vi "RNG WriteState.vi"(8 "error in (no error)":errorcluster, 10 "State":u64, 11 "RNG in":refnum<class "RNG.lvclass">) -> (0 "error out":errorcluster, 3 "RNG out":refnum<class "RNG.lvclass">)   [LabVIEW 2020, in "OpenLvVision_OpenCv.lvlib" / "RNG.lvclass"]
doc: "Write the state to the rng object."
uses:
  RNG.lvclass
  _LvHelpers/EdvrObject/EdvrObject.lvclass
  Dlls/OlvOpenCvWrapper.dll
  C:/Users/lukas/Downloads/OpenLvVision_OpenCv/SourceCode/LabView/OpenLvVision_OpenCv/_LvHelpers/EdvrObject/EdvrObject.lvclass
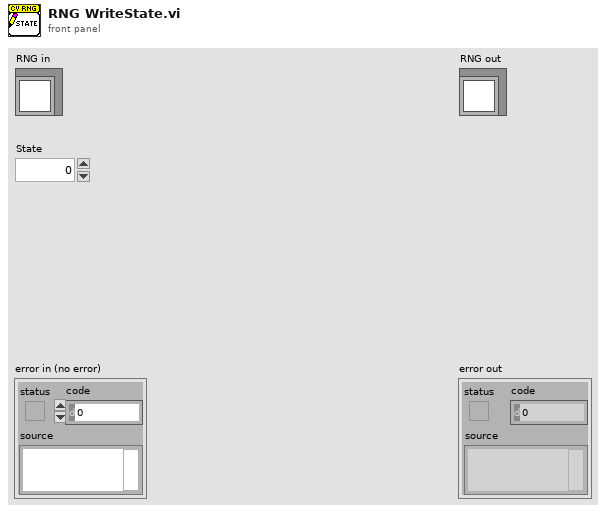
[diagram p1: front panel]
types:
  T1 = typedef "OpenLvVision_OpenCv.lvlib/EdvrObject.lvclass/Edvr.ctl" = refnum<data-value>
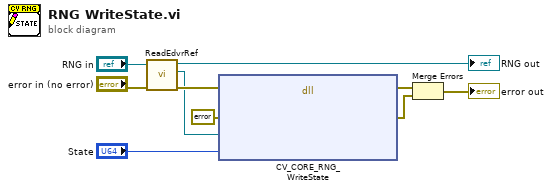
[diagram p0: block diagram]
diagram:
  n1 = call "ReadEdvrRef.vi"("error in (no error)"="error in (no error)", "EdvrObject in"="RNG in") -> ("error out"=w10:errorcluster, "Edvr"=w4:T1, "EdvrObject out"=→"RNG out":refnum<class "RNG.lvclass">)  [unwired: 7 in]
  n2 = dll-call lib="C:/Users/lukas/Downloads/OpenLvVision_OpenCv/SourceCode/LabView/OpenLvVision_OpenCv/Dlls/OlvOpenCvWrapper.dll" fn="CV_CORE_RNG_WriteState"(error in=w10, "Error"=errorcluster {"status"=FALSE, "code"=0, "source"=""} ("error constant"), "edvrRef"=w4, "state"="State") -> (error out=w8:errorcluster, "Error"=w7:errorcluster)  [unwired: 5 in, 1 out]
  n3 = Merge Errors(w8, w7) -> (→"error out":errorcluster)
